vi "ICM Config File Path.vi"(8 "error in (no error)":errorcluster) -> (0 "error out":errorcluster, 3 "ICM Config Path":path)   [LabVIEW 2015]
doc: "ICM Config File Path.vi\n\nThis VI defines where the ICM Config Files are stored.\n\nInstrument Communication Module Version 1.0\nJuly, 2017 Original Code Consulting David Thomson\n www.originalcode.com"
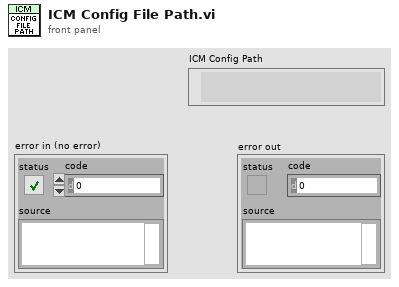
[diagram p1: front panel]
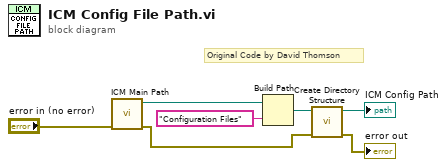
[diagram p0: block diagram]
diagram:
  # "Original Code by David Thomson"
  n1 = call "ICM Main Path.vi"("error in (no error)"="error in (no error)") -> ("error out"=w3:errorcluster, "ICM Path"=w6:path)  [unwired: 9 in]
  n2 = Build Path(base path=w6, name or relative path="Configuration Files") -> (appended path=w5:path)
  n3 = call "Create Directory Structure.vi"("error in"=w3, "Path"=w5) -> ("error out"=→"error out":errorcluster, "dup Path"=→"ICM Config Path":path)  [unwired: 4 in]
